vi "sous-VI Conversion Nombre Arabe en Nombre Romain.vi"(1 "Enter AN ARABIC NUMBER?":dbl, 2 "Roman number":bool) -> (0 "ROMAN NUMBER:":string)   [LabVIEW 2019]
panel:
  out "COMMENTAIRE:":string="entrez un nombre inferieur ou egale a 3000"
  # "Sous-VI CONVERSION NOMBRE ARABE EN NOMBRE ROMAIN:"
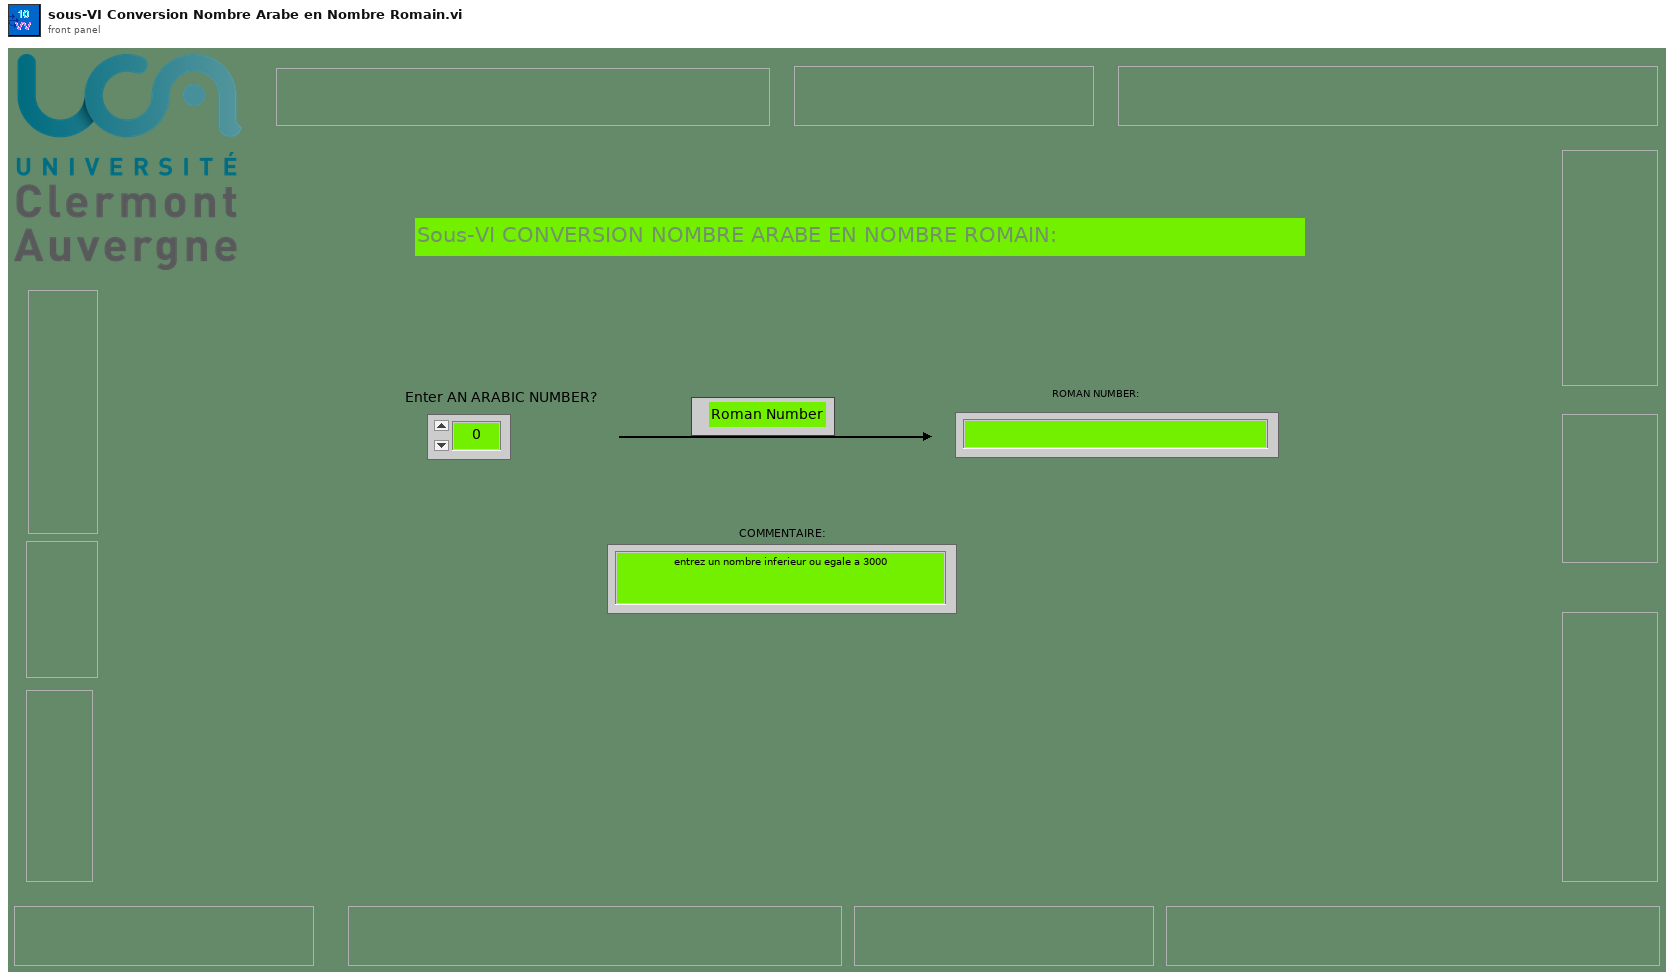
[diagram p1: front panel]
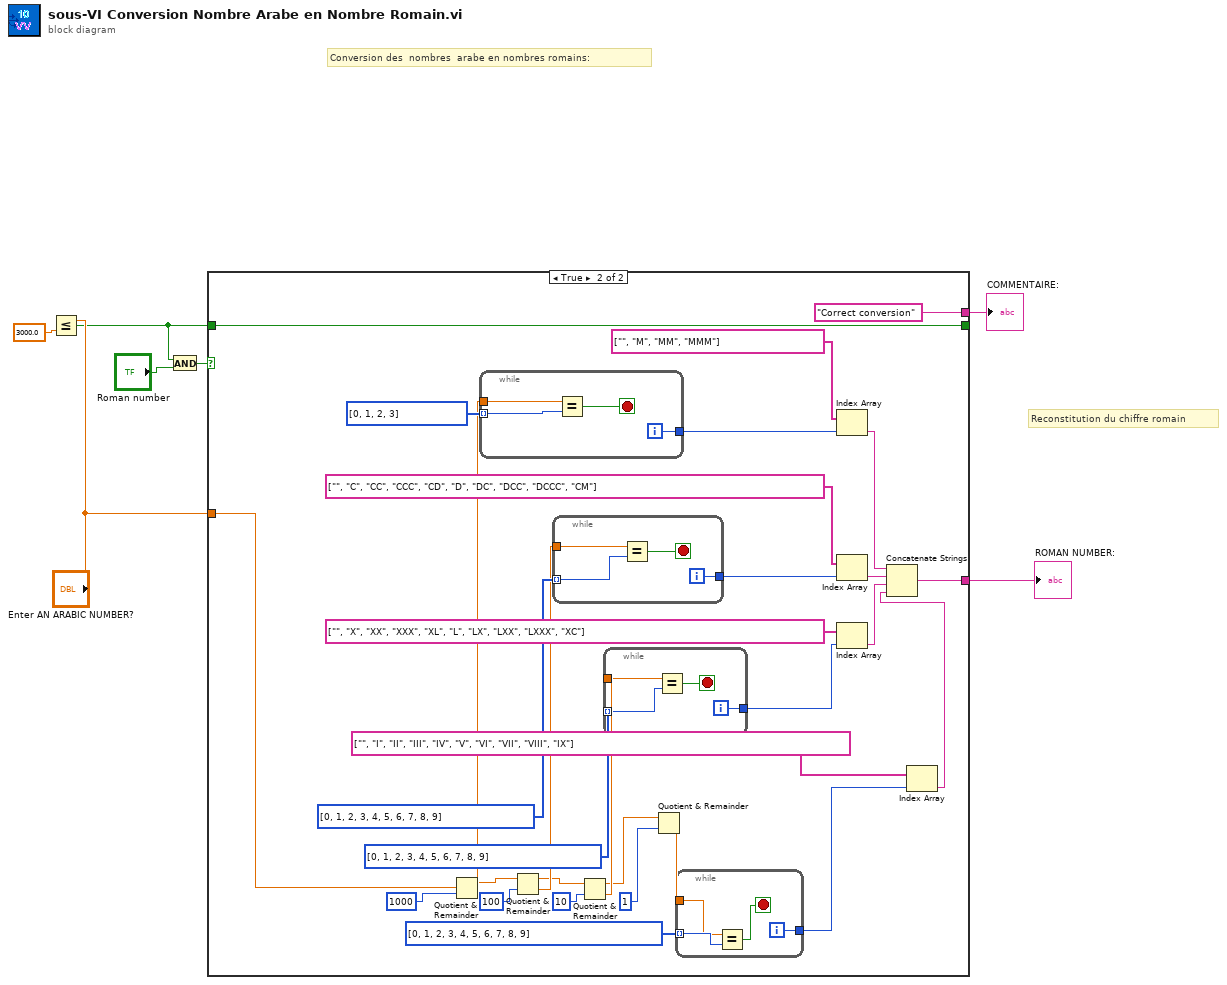
[diagram p0: block diagram]
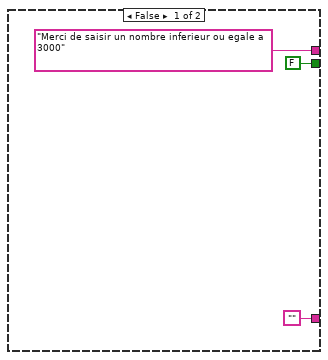
[diagram p2: hidden frame]
diagram:
  # "Reconstitution du chiffre romain"
  # "Conversion des  nombres  arabe en nombres romains:"
  n1 = Less Or Equal?(x="Enter AN ARABIC NUMBER?", y=3000.0) -> (x <= y?=w2:bool)
  n2 = And(x=w2, y="Roman number") -> (x .and. y?=w5:bool)
  n3 = case shown="True" w5 {
    tunnel: "Enter AN ARABIC NUMBER?" -> [_ w11]
    tunnel: ["Merci de saisir un nombre inferieur ou egale a 3000" "Correct conversion"] -> w3
    tunnel: w2 -> [_ w41]
    tunnel: [FALSE w41] -> _
    tunnel: ["" w12] -> w1
    frame False {
    }
    frame True {
      n4 = Quotient & Remainder(x=w11, y=1000) -> (x-y*floor(x/y)=w19:dbl, floor(x/y)=w20:dbl)
      n5 = while {
        tunnel: i32[] [0, 1, 2, 3] -> [w57] mode=indexing
        tunnel: [w56] -> w38
        tunnel: w20 -> [w55]
        i -> [w56]
        stop <- w54 stop-if-true
        n6 = Equal?(x=w55, y=w57) -> (x = y?=w54:bool)
      }
      n7 = Quotient & Remainder(x=w19, y=100) -> (x-y*floor(x/y)=w17:dbl, floor(x/y)=w18:dbl)
      n8 = while {
        tunnel: i32[] [0, 1, 2, 3, 4, 5, 6, 7, 8, 9] -> [w49] mode=indexing
        tunnel: [w48] -> w32
        tunnel: w18 -> [w47]
        i -> [w48]
        stop <- w46 stop-if-true
        n9 = Equal?(x=w47, y=w49) -> (x = y?=w46:bool)
      }
      n10 = Quotient & Remainder(x=w17, y=10) -> (x-y*floor(x/y)=w15:dbl, floor(x/y)=w16:dbl)
      n11 = while {
        tunnel: i32[] [0, 1, 2, 3, 4, 5, 6, 7, 8, 9] -> [w53] mode=indexing
        tunnel: [w52] -> w35
        tunnel: w16 -> [w51]
        i -> [w52]
        stop <- w50 stop-if-true
        n12 = Equal?(x=w51, y=w53) -> (x = y?=w50:bool)
      }
      n13 = Quotient & Remainder(x=w15, y=1) -> (floor(x/y)=w21:dbl)  [unwired: 1 out]
      n14 = while {
        tunnel: i32[] [0, 1, 2, 3, 4, 5, 6, 7, 8, 9] -> [w45] mode=indexing
        tunnel: [w44] -> w30
        tunnel: w21 -> [w43]
        i -> [w44]
        stop <- w42 stop-if-true
        n15 = Equal?(x=w43, y=w45) -> (x = y?=w42:bool)
      }
      n16 = Index Array(array=string[] ["", "M", "MM", "MMM"], index=w38) -> (element=w29:string)
      n17 = Index Array(array=string[] ["", "C", "CC", "CCC", "CD", "D", "DC", "DCC", "DCCC", "CM"], index=w32) -> (element=w27:string)
      n18 = Index Array(array=string[] ["", "X", "XX", "XXX", "XL", "L", "LX", "LXX", "LXXX", "XC"], index=w35) -> (element=w28:string)
      n19 = Index Array(array=string[] ["", "I", "II", "III", "IV", "V", "VI", "VII", "VIII", "IX"], index=w30) -> (element=w26:string)
      n20 = Concatenate Strings(w29, w27, w28, w26) -> (w12:string)
    }
  }
  "COMMENTAIRE:" <- w3
  "ROMAN NUMBER:" <- w1
